vi "DataType Cacher(Data).vi"(7 "GroupName(\"\")":string, 8 "error in (no error)":errorcluster, 9 "Data":variant, 10 "key(use dataname if empty)":string) -> (0 "error out":errorcluster, 1 "Data(Dup)":variant, 2 "stored type":T1, 3 "match?":bool, 6 "cacher":variant)   [LabVIEW 2017]
uses:
  <vilib>/Utility/Data Type/Type Definitions/Data Type.ctl
  <vilib>/Utility/Data Type/NI_Data Type.lvlib
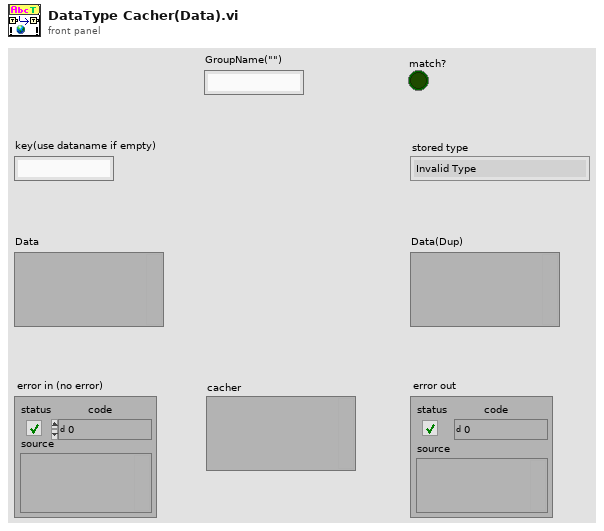
[diagram p1: front panel]
types:
  T1 = typedef "NI_Data Type.lvlib/Data Type.ctl" = enum8{"Invalid Type", "Void", "I8", "I16", "I32", "I64", "U8", "U16", "U32", "U64", "Single Float", "Double Float", "Extended Float", "Single Complex", "Double Complex", "Extended Complex", "Enum U8", "Enum U16", "Enum U32", "Enum U64", "Single Float With Unit", "Double Float With Unit", "Extended Float With Unit", "Single Complex with Unit", "Double Complex with Unit", "Extended Complex with Unit", "Boolean", "String", "Path", "Picture", "Tag", "Array", "Cluster", "Variant", "LV Variant", "Waveform", "Timestamp", "Digital Waveform", "Digital Data", "ExpressData", "Refnum", "External Data", "VI", "Poly VI", "LabVIEW Class Instance", "Fixed Point"}
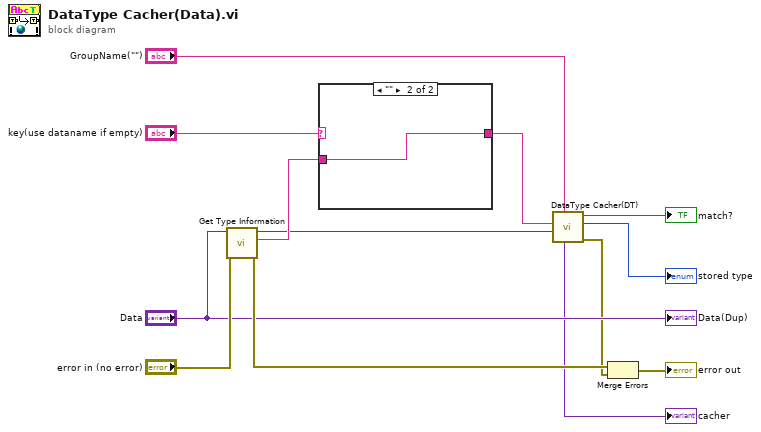
[diagram p0: block diagram]
diagram:
  n1 = call <vilib>:"Get Type Information.vi"("error in (no error)"="error in (no error)", "Variant"="Data") -> ("error out"=w12:errorcluster, "Name"=w9:string, "Type"=w3:T1)  [unwired: 5 in, 2 out]
  n2 = case shown="\"\"" "key(use dataname if empty)" {
    selector: "key(use dataname if empty)" -> [w14 _]
    tunnel: w9 -> [_ w15]
    tunnel: [w14 w15] -> w8
    frame "False", Default {
    }
    frame "" {
    }
  }
  n3 = call "DataType Cacher(DT).vi"("GroupName(\"\")"="GroupName(\"\")", "Type"=w3, "key"=w8) -> ("error out"=w5:errorcluster, "stored type"=→"stored type":T1, "match?"=→"match?":bool, "cacher"=→"cacher":variant)  [unwired: 5 in]
  n4 = Merge Errors(w12, w5) -> (→"error out":errorcluster)
  "Data(Dup)" <- "Data"
